vi "Write Built Export's Full Path.vi"(8 "error in (no error)":errorcluster, 10 "Built Export's Full Path":path, 11 "Export in":refnum<class "Export.lvclass">) -> (0 "error out":errorcluster, 3 "Export out":refnum<class "Export.lvclass">)   [LabVIEW 2017, in "CL_G3_VIComponentBuilder.lvlib" / "Export.lvclass"]
uses:
  Export.lvclass
  Export.lvclass/Export.ctl
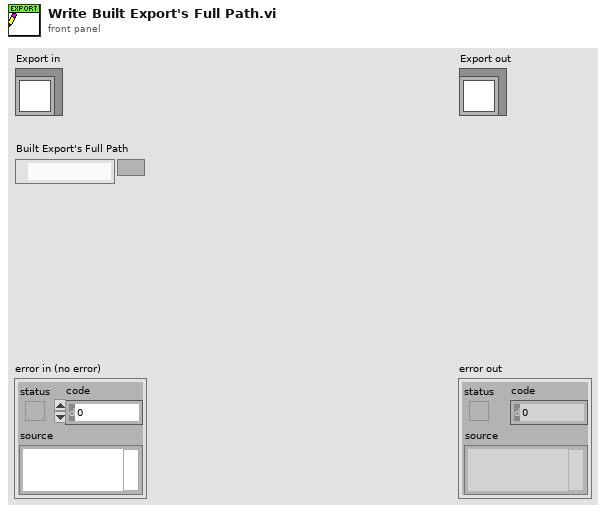
[diagram p1: front panel]
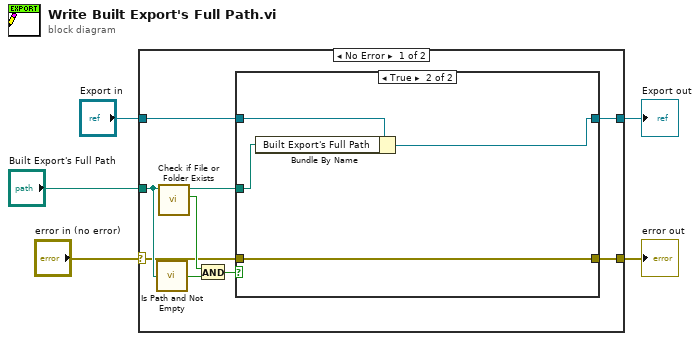
[diagram p0: block diagram]
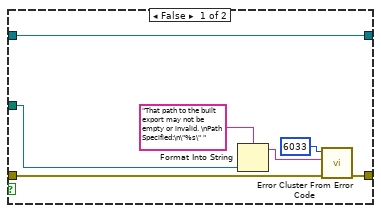
[diagram p2: hidden frame]
diagram:
  n1 = case shown="No Error" "error in (no error)" {
    selector: "error in (no error)" -> [w7 w26]
    tunnel: [w6 w26] -> w4
    tunnel: [w13 w27] -> w2
    tunnel: "Export in" -> [w14 w27]
    tunnel: "Built Export's Full Path" -> [w11 _]
    frame No Error {
      n2 = call <vilib>:"Is Path and Not Empty.vi"("path"=w11) -> ("Is Path and Not Empty?"=w10:bool)  [unwired: 4 in]
      n3 = call <vilib>:"Check if File or Folder Exists.vi"("path"=w11) -> ("file or folder exists?"=w9:bool, "dup path"=w12:path)  [unwired: 8 in, 1 out]
      n4 = And(x=w9, y=w10) -> (x .and. y?=w8:bool)
      n5 = case shown="True" w8 {
        tunnel: w14 -> [w21 w25]
        tunnel: [w21 w24] -> w13
        tunnel: w12 -> [w19 w23]
        tunnel: w7 -> [w17 w22]
        tunnel: [w16 w22] -> w6
        frame False {
          n6 = Format Into String(format string="That path to the built export may not be empty or invalid. \nPath Specified:\n\"%s\" " ("source"), w19) -> (resulting string=w18:string)  [unwired: 2 in, 1 out]
          n7 = call <vilib>:"Error Cluster From Error Code.vi"("error in (no error)"=w17, "error message (\"\")"=w18, "error code (0)"=6033) -> ("error out"=w16:errorcluster)  [unwired: 6 in]
        }
        frame True {
          n8 = Bundle By Name(cluster=w25, "Built Export's Full Path"=w23) -> (w24:refnum<class "Export.lvclass">)
        }
      }
    }
    frame Error {
    }
  }
  "error out" <- w4
  "Export out" <- w2
